vi "oa_TV Calculate Continuous Angular Speed (1Chan).vi"(6 "pulse/revolution (1)":i32=1, 7 "reset? (False)":bool, 8 "error in (no error)":errorcluster, 9 "filter coefficients":dbl[](array[numeric])=[1.0, 1.0, 1.0] format="%.2f", 10 "deltaX":dbl, 11 "Y[n]":dbl[](array[numeric])=[1.0, 2.0, 3.0]) -> (0 "error out":errorcluster, 2 "dY[n]/dX[n]":dbl[](array[numeric])=[3.0, 6.0, 9.0] format="%.2f", 3 "pulse out":dbl[](array[numeric])=[1.0, 2.0, 3.0] format="%.2f")   [LabVIEW 2017, in "SoundVib_Torsional.lvlib"]
uses:
  <vilib>/addons/Sound and Vibration/Order Analysis/Torsional Vibration/SoundVib_Torsional.lvlib
  <vilib>/Analysis/3filter.llb/FIR Filter with I.C. (DBL).vi
  <vilib>/Analysis/NI_AALBase.lvlib
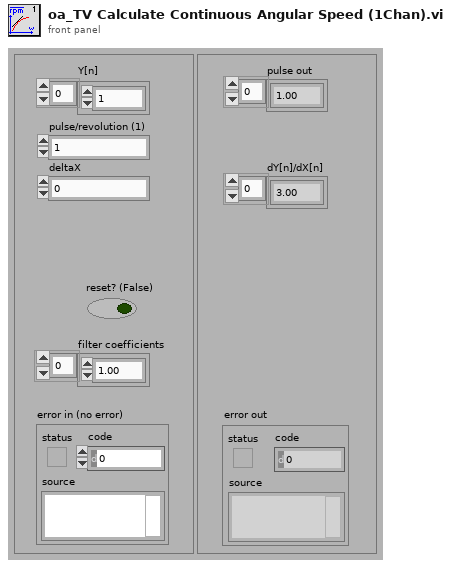
[diagram p1: front panel]
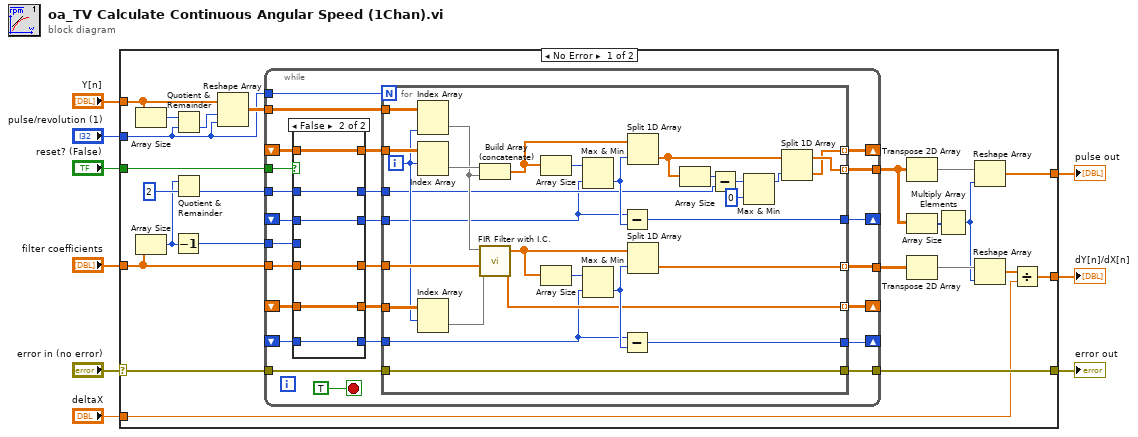
[diagram p0: block diagram]
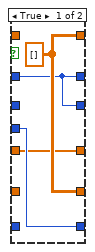
[diagram p2: hidden frame]
diagram:
  n1 = case shown="No Error" "error in (no error)" {
    selector: "error in (no error)" -> [w32 w97]
    tunnel: [w19 w97] -> w1
    tunnel: [w16 _] -> w2
    tunnel: [w23 _] -> w3
    tunnel: "Y[n]" -> [w29 _]
    tunnel: "reset? (False)" -> [w31 _]
    tunnel: "pulse/revolution (1)" -> [w15 _]
    tunnel: "deltaX" -> [w18 _]
    tunnel: "filter coefficients" -> [w10 _]
    frame No Error {
      n2 = Array Size(array=w29) -> (size(s)=w30:i32)
      n3 = Array Size(array=w10) -> (size(s)=w13:i32)
      n4 = Decrement(x=w13) -> (x-1=w11:i32)
      n5 = Quotient & Remainder(x=w30, y=w15) -> (floor(x/y)=w28:i32)  [unwired: 1 out]
      n6 = Quotient & Remainder(x=w13, y=2) -> (floor(x/y)=w12:i32)  [unwired: 1 out]
      n7 = Reshape Array(w29, w28, w15) -> (w27:dbl[][])
      n8 = while {
        tunnel: [w48] -> w20
        tunnel: w32 -> [w45]
        tunnel: w10 -> [w37]
        shift-right: [w46] -> _
        shift-left: _ -> [w55]
        shift-right: [w52] -> _
        shift-left: _ -> [w56]
        shift-right: [w49] -> _
        shift-left: _ -> [w39]
        tunnel: w31 -> [w38]
        tunnel: [w51] -> w25
        shift-right: [w47] -> _
        shift-left: _ -> [w41]
        tunnel: w15 -> [w53]
        tunnel: w27 -> [w50]
        tunnel: [w44] -> w19
        tunnel: w12 -> [w34]
        tunnel: w11 -> [w33]
        stop <- TRUE stop-if-true
        n9 = case shown="False" w38 {
          tunnel: w56 -> [_ w67]
          tunnel: w55 -> [_ w65]
          tunnel: [w60 w67] -> w54
          tunnel: [w60 w65] -> w43
          tunnel: [w61 w64] -> w42
          tunnel: w41 -> [_ w64]
          tunnel: w33 -> [w61 _]
          tunnel: w34 -> [w58 w62]
          tunnel: [w58 w66] -> w40
          tunnel: w39 -> [_ w66]
          tunnel: w37 -> [w59 w63]
          tunnel: [w59 w63] -> w36
          tunnel: [w58 w62] -> w35
          frame True {
            w60 = dbl[][] [] ("Array")
          }
          frame False {
          }
        }
        n10 = for {
          N: w53 -> [_]
          tunnel: [w69] -> w48 mode=indexing
          tunnel: w45 -> [w74]
          tunnel: w36 -> [w78]
          tunnel: [w94] -> w49
          tunnel: [w90] -> w51 mode=indexing
          tunnel: [w87] -> w47
          tunnel: w54 -> [w83]
          tunnel: [w84] -> w52 mode=indexing
          tunnel: w43 -> [w81]
          tunnel: w50 -> [w80]
          tunnel: [w76] -> w46 mode=indexing
          tunnel: [w74] -> w44
          tunnel: w42 -> [w72]
          tunnel: w35 -> [w71]
          tunnel: w40 -> [w70]
          i -> [w73]
          n11 = Index Array(array=w80, index (col)=w73) -> (element=w79:dbl[])  [unwired: 1 in]
          n12 = Index Array(array=w83, index (row)=w73) -> (element=w82:dbl[])  [unwired: 1 in]
          n13 = Index Array(array=w81, index (row)=w73) -> (element=w75:dbl[])  [unwired: 1 in]
          n14 = Build Array (concatenate)(w82, w79) -> (w85:dbl[])
          n15 = call-poly <vilib>:"FIR Filter with I.C..vi"("Initial X Conditions"=w75, "FIR Coefficients"=w78, "X"=w79) -> ("Final X Conditions"=w76:dbl[], "Filtered X"=w77:dbl[])  [unwired: 5 in, 1 out]
          n16 = Array Size(array=w85) -> (size(s)=w96:i32)
          n17 = Array Size(array=w77) -> (size(s)=w89:i32)
          n18 = Max & Min(x=w96, y=w70) -> (min(x,y)=w95:i32)  [unwired: 1 out]
          n19 = Max & Min(x=w89, y=w72) -> (min(x,y)=w88:i32)  [unwired: 1 out]
          n20 = Subtract(x=w70, y=w95) -> (x-y=w94:i32)
          n21 = Subtract(x=w72, y=w88) -> (x-y=w87:i32)
          n22 = Split 1D Array(array=w85, index=w95) -> (second subarray=w68:dbl[])  [unwired: 1 out]
          n23 = Split 1D Array(array=w77, index=w88) -> (second subarray=w69:dbl[])  [unwired: 1 out]
          n24 = Array Size(array=w68) -> (size(s)=w93:i32)
          n25 = Subtract(x=w93, y=w71) -> (x-y=w92:i32)
          n26 = Max & Min(x=w92, y=0) -> (max(x,y)=w86:i32)  [unwired: 1 out]
          n27 = Split 1D Array(array=w68, index=w86) -> (first subarray=w90:dbl[], second subarray=w84:dbl[])
        }
      }
      n28 = Transpose 2D Array(2D array=w25) -> (transposed array=w26:dbl[][])
      n29 = Array Size(array=w25) -> (size(s)=w24:i32[])
      n30 = Transpose 2D Array(2D array=w20) -> (transposed array=w22:dbl[][])
      n31 = Multiply Array Elements(1:w24) -> (0:w21:i32)
      n32 = Reshape Array(w26, w21) -> (w23:dbl[])
      n33 = Reshape Array(w22, w21) -> (w17:dbl[])
      n34 = Divide(x=w17, y=w18) -> (x/y=w16:dbl[])
    }
    frame Error {
    }
  }
  "dY[n]/dX[n]" <- w2
  "error out" <- w1
  "pulse out" <- w3
